vi "G#Debugger_Refresh.vi"(0 "Objects dvr":refnum<data-value>, 1 "full class name":string, 5 "error in (no error)":errorcluster) -> (19 "error out":errorcluster)   [LabVIEW 2017, in "G#Debugger.lvlib"]
uses:
  <vilib>/addons/_AddQ/G#Debugger/G#Debugger.lvlib
  <vilib>/addons/_AddQ/G#Object/utils/G#Object_ClassInfoType.ctl
  <vilib>/addons/_AddQ/G#Object/G#Object.lvclass
  <vilib>/addons/_AddQ/G#Object/utils/G#Object_ObjectInfoType.ctl
  <vilib>/addons/_AddQ/G#Object/utils/G#Object_CreateMethod.ctl
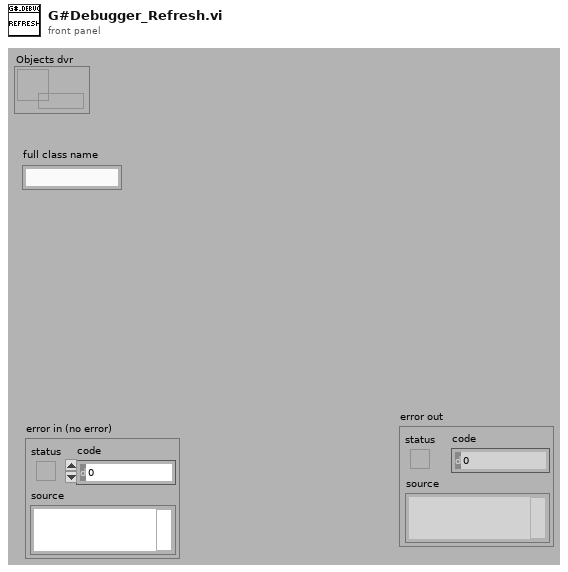
[diagram p1: front panel]
types:
  T1 = typedef "G#Object.lvclass/G#Object_ClassInfoType.ctl" = cluster{"ClassName":string, "ObjectInfo":T2[], "ObjectRefs":refnum<class "G#Object.lvclass">[], "TypeRef":refnum<class "G#Object.lvclass">}
  T2 = typedef "G#Object.lvclass/G#Object_ObjectInfoType.ctl" = cluster{"ObjectName":string, "ObjectID":u32, "Users":i32, "Counter":bool, "AttributeRefs":u32[], "FullClassName":string, "ClassName":string, "CreateMethod":T3, "GenericDestructorExists":bool, "Owner":string}
  T3 = typedef "G#Object.lvclass/G#Object_CreateMethod.ctl" = enum16{"Create", "Create or look up existing", "Look up existing"}
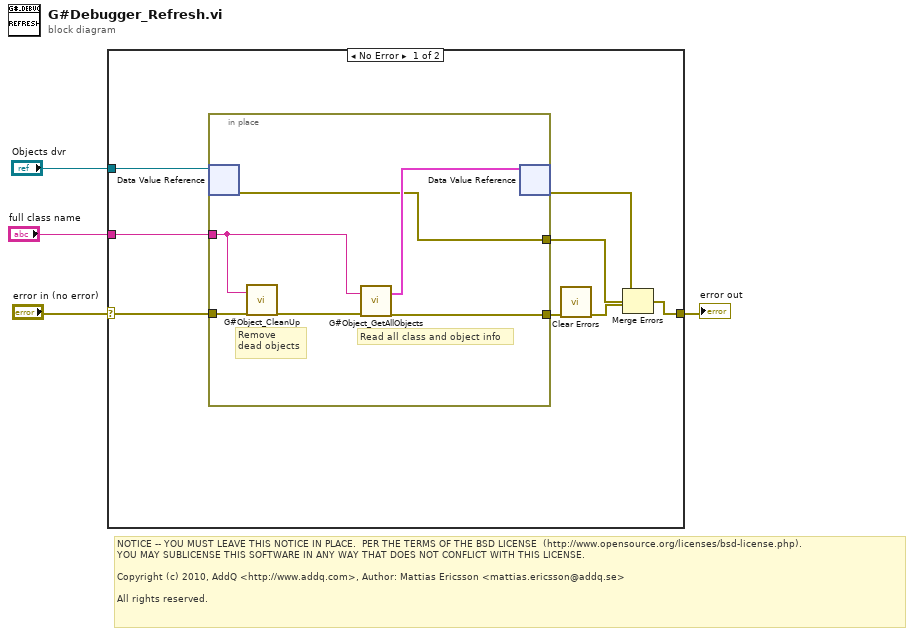
[diagram p0: block diagram]
diagram:
  # "NOTICE -- YOU MUST LEAVE THIS NOTICE IN PLACE.  PER THE TERMS OF THE BSD LICENSE  (http://www.opensource.org/licenses/bsd-license.php).\nYOU MAY SUBLICENSE THIS SOFTWARE IN ANY WAY THAT DOES NOT CONFLICT WITH THIS LICENSE.\n\nCopyright (c) 2010, AddQ <http://www.addq.com>, Author: Mattias Ericsson <mattias.ericsson@addq.se>\n\nAll rights reserved."
  n1 = case shown="No Error" "error in (no error)" {
    selector: "error in (no error)" -> [w12 w19]
    tunnel: [w9 w19] -> w3
    tunnel: "Objects dvr" -> [w11 _]
    tunnel: "full class name" -> [w10 _]
    frame No Error {
      n2 = in-place {
        in-place-border: w12 -> [w15]
        in-place-border: w10 -> [w13]
        in-place-border: [w17] -> w6
        in-place-border: [w16] -> w7
        # "Read all class and object info"
        # "Remove\ndead objects"
        n3 = in-place-dvr #1(w11) -> (w16:errorcluster)  [unwired: 1 out]
        n4 = call <vilib>:"G#Object_CleanUp.vi"("full class name (\"\")"=w13, "error in (no error)"=w15) -> ("error out"=w14:errorcluster)  [unwired: 16 in, 1 out]
        n5 = call <vilib>:"G#Object_GetAllObjects.vi"("full class name (\"\")"=w13, "error in (no error)"=w14) -> ("class information"=w18:T1[], "error out"=w17:errorcluster)  [unwired: 14 in, 2 out]
        n6 = in-place-dvr #1(w18) -> (w8:errorcluster)  [unwired: 1 out]
      }
      n7 = call <vilib>:"Clear Errors.vi"("error in (no error)"=w6) -> ("error out"=w5:errorcluster)  [unwired: 5 in, 1 out]
      n8 = Merge Errors(w8, w7, w5) -> (w9:errorcluster)
    }
    frame Error {
    }
  }
  "error out" <- w3
